vi "Ginzburg-Levanyuk.vi"() -> ()   [LabVIEW 2021]
panel:
  out "Epsilon from k":dbl
  out "Gi Si":dbl format="%#_6e"
  out "Gi Gurevich":dbl format="%#_6e"
  in  "k GL":dbl
  out "Lambda ab0":dbl format="%#_6p"
  in  "delta C":dbl=13.0
  out "Eps ab0":dbl format="%#_6p"
  in  "B'c2":dbl
  out "Gi larkin":dbl
  out "Gi Koshelev":dbl format="%#_6e"
  in  "epcilon":dbl format="%#_6p"
  in  "Lambda":dbl format="%#_6p"
  in  "Tc":dbl
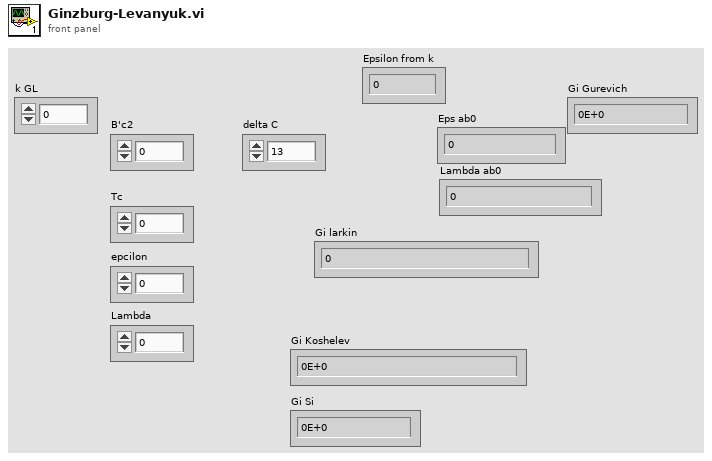
[diagram p1: front panel]
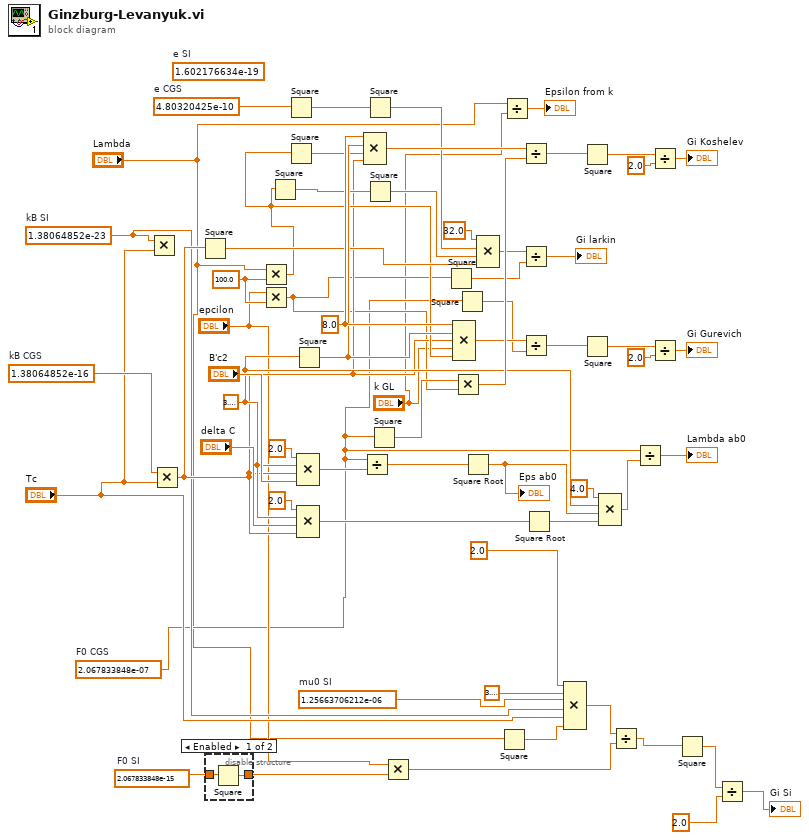
[diagram p0: block diagram]
diagram:
  w6 = 1.25663706212e-06  # mu0 SI
  w30 = 1.38064852e-16  # kB CGS
  w18 = 1.38064852e-23  # kB SI
  (unwired) 1.602176634e-19  # e SI
  w23 = 4.80320425e-10  # e CGS
  w57 = 100.0 ("y")
  w5 = 2.067833848e-07  # F0 CGS
  w14 = 2.067833848e-15  # F0 SI
  w38 = 8.0
  w44 = 3.141592653589793
  n1 = Multiply(x=w18, y="Tc") -> ()  [unwired: 1 out]
  n2 = Multiply(x=w30, y="Tc") -> (x*y=w21:dbl)
  n3 = Square(x=w21) -> (x^2=w27:dbl)
  n4 = disable-structure shown="Enabled" {
    disable-tunnel: w14 -> [w65 w66]
    disable-tunnel: [w64 w66] -> w4
    frame Enabled {
      n5 = Square(x=w65) -> (x^2=w64:dbl)
    }
    frame Disabled {
    }
  }
  n6 = Multiply(x="Lambda", y=w57) -> (x*y=w22:dbl)
  n7 = Multiply(x="epcilon", y=w57) -> (x*y=w20:dbl)
  n8 = Square(x=w22) -> (x^2=w26:dbl)
  n9 = Square(x=w23) -> (x^2=w56:dbl)
  n10 = Square(x=w22) -> (x^2=w25:dbl)
  n11 = Square(x=w44) -> (x^2=w37:dbl)
  n12 = Compound Arithmetic op=MULTIPLY(2.0, w44, w21, "B'c2") -> (w49:dbl)
  n13 = Compound Arithmetic op=MULTIPLY(2.0, w44, "delta C", w21) -> (w42:dbl)
  n14 = Divide(x=w5, y=w49) -> (x/y=w48:dbl)
  n15 = Compound Arithmetic op=MULTIPLY(w38, w37, w25, w21) -> (w63:dbl)
  n16 = Square(x=w56) -> (x^2=w29:dbl)
  n17 = Square(x=w26) -> (x^2=w28:dbl)
  n18 = Square(x=w5) -> (x^2=w53:dbl)
  n19 = Multiply(x="epcilon", y=w4) -> (x*y=w12:dbl)
  n20 = Square(x=w20) -> (x^2=w24:dbl)
  n21 = Compound Arithmetic op=MULTIPLY(w38, w37, w21, "k GL", w22) -> (w36:dbl)
  n22 = Multiply(x=w53, y=w20) -> (x*y=w62:dbl)
  n23 = Square(x=w5) -> (x^2=w35:dbl)
  n24 = Square Root(x=w48) -> (sqrt(x)=w46:dbl)
  "Eps ab0" <- w46
  n25 = Compound Arithmetic op=MULTIPLY(32.0, w29, w28, w27) -> (w54:dbl)
  n26 = Square(x="Lambda") -> (x^2=w16:dbl)
  n27 = Divide(x="Lambda", y="k GL") -> (x/y=→"Epsilon from k":dbl)
  n28 = Divide(x=w63, y=w62) -> (x/y=w61:dbl)
  n29 = Divide(x=w54, y=w24) -> (x/y=→"Gi larkin":dbl)
  n30 = Divide(x=w36, y=w35) -> (x/y=w34:dbl)
  n31 = Square Root(x=w42) -> (sqrt(x)=w41:dbl)
  n32 = Compound Arithmetic op=MULTIPLY(2.0, 3.141592653589793, w6, w18, "Tc", w16) -> (w15:dbl)
  n33 = Square(x=w61) -> (x^2=w60:dbl)
  n34 = Square(x=w34) -> (x^2=w33:dbl)
  n35 = Compound Arithmetic op=MULTIPLY(4.0, w44, w46, w41) -> (w40:dbl)
  n36 = Divide(x=w15, y=w12) -> (x/y=w11:dbl)
  n37 = Divide(x=w5, y=w40) -> (x/y=→"Lambda ab0":dbl)
  n38 = Divide(x=w60, y=2.0) -> (x/y=→"Gi Koshelev":dbl)
  n39 = Divide(x=w33, y=2.0) -> (x/y=→"Gi Gurevich":dbl)
  n40 = Square(x=w11) -> (x^2=w10:dbl)
  n41 = Divide(x=w10, y=2.0) -> (x/y=→"Gi Si":dbl)
